vi "ConstructorString.vi"(6 "error in":errorcluster, 9 "WhileLoop in":refnum<class "WhileLoop.lvclass">) -> (0 "error out":errorcluster, 3 "WhileLoop out":refnum<class "WhileLoop.lvclass">, 4 "constructor":string)   [LabVIEW 2014, in "Raspberry Pi Compatible Compiler for LabVIEW.lvlib" / "WhileLoop.lvclass"]
uses:
  WhileLoop.lvclass
  WhileLoop.lvclass/WhileLoop.ctl
  Python/Parsing/ListTypesTD.ctl
  Python/Parsing/Python Functions.lvlib
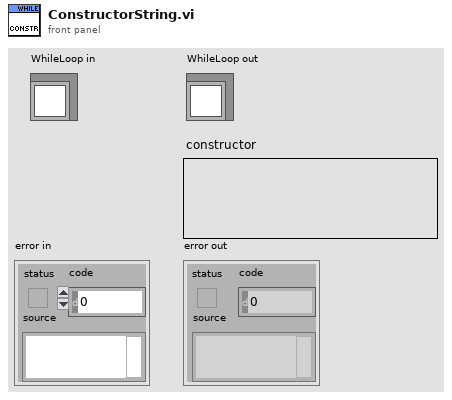
[diagram p1: front panel]
types:
  T1 = typedef "Raspberry Pi Compatible Compiler for LabVIEW.lvlib/Python Functions.lvlib/ListTypesTD.ctl" = enum16{"list", "tuple", "parameter list", "output list", "return values"}
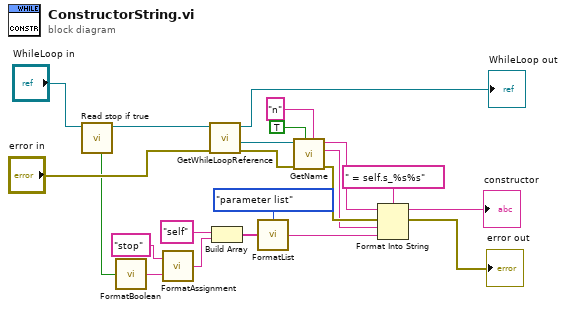
[diagram p0: block diagram]
diagram:
  n1 = call "Read stop if true.vi"("ForLoop in"="WhileLoop in") -> ("ForLoop out"=w6:refnum<class "WhileLoop.lvclass">, "stop if true"=w4:bool)  [unwired: 7 in]
  n2 = call "FormatBoolean.vi"("value"=w4) -> ("python object"=w9:string)
  n3 = call "FormatAssignment.vi"("value"=w9, "name"="stop") -> ("python assignment"=w2:string)
  n4 = call "GetWhileLoopReference.vi"("error in"="error in", "WhileLoop in"=w6) -> ("error out"=w14:errorcluster, "reference out"=w15:refnum<vi>, "WhileLoop out"=→"WhileLoop out":refnum<class "WhileLoop.lvclass">)  [unwired: 7 in]
  n5 = Build Array("self" ("String"), w2) -> (w1:string[])
  n6 = call "FormatList.vi"("values"=w1, "type"=ListTypesTD."parameter list") -> ("python object"=w20:string)
  n7 = call "GetName.vi"("base name"="n", "add self"=TRUE, "error in"=w14, "GObj Refnum"=w15) -> ("error out"=w13:errorcluster, "UID"=w10:string, "name"=w11:string)  [unwired: 5 in]
  n8 = Format Into String(format string=" = self.s_%s%s", initial string=w11, error in=w13, w10, w20) -> (resulting string=→"constructor":string, error out=→"error out":errorcluster)
